vi "Current Channels Array.vi"(0 "Channel 1":string, 5 "Relays Array In":bool[](array[boolean])=[FALSE, FALSE, FALSE, FALSE, FALSE, FALSE, FALSE, FALSE, FALSE, FALSE, FALSE, FALSE, FALSE, FALSE, FALSE, FALSE, FALSE, FALSE, FALSE, FALSE, FALSE, FALSE, FALSE, FALSE, FALSE, FALSE, FALSE, FALSE, FALSE, FALSE, FALSE, FALSE, FALSE, FALSE, FALSE, FALSE, FALSE, FALSE, FALSE, FALSE, FALSE, FALSE, FALSE, FALSE, FALSE, FALSE, FALSE, FALSE, FALSE, FALSE, FALSE, FALSE, FALSE, FALSE, FALSE, FALSE, FALSE, FALSE, FALSE, FALSE, FALSE, FALSE, FALSE, FALSE, FALSE, FALSE, FALSE, FALSE, FALSE, FALSE, FALSE, FALSE, FALSE, FALSE, FALSE, FALSE, FALSE, FALSE, FALSE, FALSE, FALSE, FALSE, FALSE, FALSE, FALSE, FALSE, FALSE, FALSE, FALSE, FALSE, FALSE, FALSE, FALSE, FALSE, FALSE, FALSE], 7 "N shift to Min Channel Current":u32, 9 "Range and Function":T1(ring), 11 "error in":errorcluster, 13 "State":bool) -> (4 "Current Channel?":bool, 6 "Relay Array out":bool[](array[boolean]), 15 "error out":errorcluster)   [LabVIEW 2021, in "DMM_Scan DAQ Ext RLY.lvlib"]
doc: "Checks if Channel 1 from the Scan List is a current channel and will Open/Close the corresponding Shunt Relay in the Relay Array."
uses:
  DMM_Scan DAQ Ext RLY.lvlib
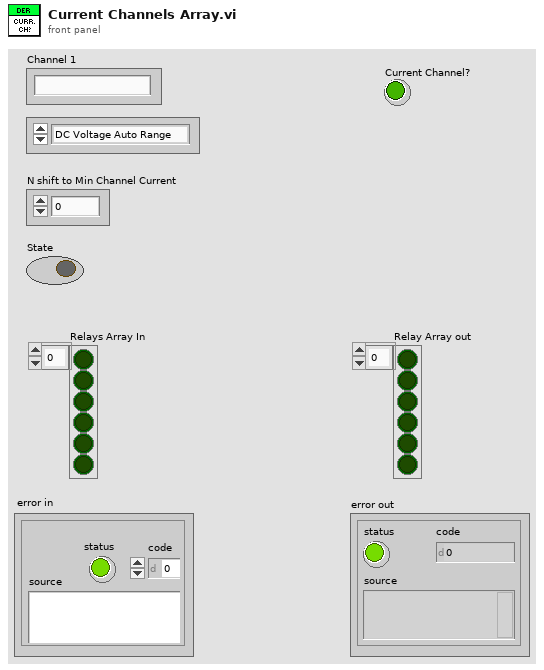
[diagram p1: front panel]
types:
  T1 = enum16{"DC Voltage Auto Range", "DC 100 mV", "DC 1 V ", "DC 10 V", "DC 100 V", "DC 300 V", " ", "AC Voltage Auto Range", "AC 50 mV", "AC 200 mV", "AC 500 mV", "AC 2 V", "AC 5 V", "AC 20 V", "AC 50 V", "AC 300 V", "  ", "DC Current Auto Range", "DC 1 uA", "DC 10 uA", "DC 100 uA", "DC 1 mA", "DC 10 mA", "DC 20 mA", "DC 100 mA", "DC 200 mA", "DC 1 A", "DC 3 A", "   ", "AC Current Auto Range", "AC 100 uA", "AC 1 mA", "AC 10 mA", "AC 100 mA", "AC 500 mA", "AC 1 A", "AC 3 A", "    ", "Resistance Auto Range", "Res 100 Ohm", "Res 1 kOhm", "Res 10 kOhm", "Res 100 kOhm", "Res 1 MOhm", "Res 10 MOhm", "Res 100 MOhm", "Res 5 GOhm", "     ", "Frequency AC Auto Range", "Freq AC 50 mV", "Freq AC 500 mV", "Freq AC 5 V", "Freq AC 50 V", "Freq AC 300 V", "      ", "Period AC Auto Range", "Period AC 50 mV", "Period AC 500 mV", "Period AC 5 V", "Period AC 50 V", "Period AC 300 V"}
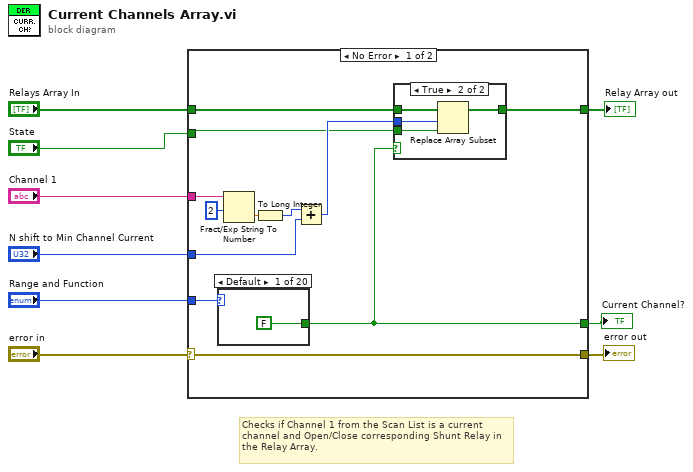
[diagram p0: block diagram]
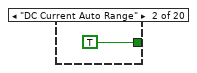
[diagram p3: hidden frame]
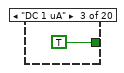
[diagram p4: hidden frame]
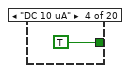
[diagram p5: hidden frame]
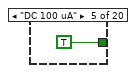
[diagram p6: hidden frame]
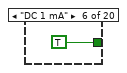
[diagram p7: hidden frame]
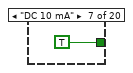
[diagram p8: hidden frame]
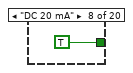
[diagram p9: hidden frame]
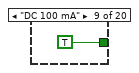
[diagram p10: hidden frame]
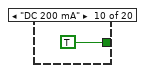
[diagram p11: hidden frame]
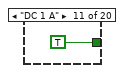
[diagram p12: hidden frame]
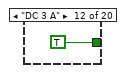
[diagram p13: hidden frame]
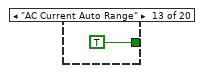
[diagram p14: hidden frame]
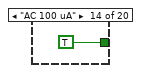
[diagram p15: hidden frame]
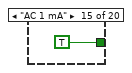
[diagram p16: hidden frame]
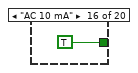
[diagram p17: hidden frame]
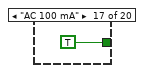
[diagram p18: hidden frame]
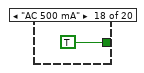
[diagram p19: hidden frame]
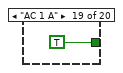
[diagram p20: hidden frame]
diagram:
  # "Checks if Channel 1 from the Scan List is a current channel and Open/Close corresponding Shunt Relay in the Relay Array."
  n1 = case shown="No Error" "error in" {
    selector: "error in" -> [w19 w49]
    tunnel: "Channel 1" -> [w17 _]
    tunnel: [w19 w49] -> w7
    tunnel: [w10 FALSE] -> w6
    tunnel: "N shift to Min Channel Current" -> [w16 _]
    tunnel: "Relays Array In" -> [w13 w47]
    tunnel: [w15 w47] -> w3
    tunnel: "State" -> [w12 _]
    tunnel: "Range and Function" -> [w11 _]
    frame No Error {
      n2 = case shown="Default" w11 {
        tunnel: [FALSE TRUE TRUE TRUE TRUE TRUE TRUE TRUE TRUE TRUE TRUE TRUE TRUE TRUE TRUE TRUE TRUE TRUE TRUE TRUE] -> w10
        frame Default {
        }
        frame "DC Current Auto Range" {
        }
        frame "DC 1 uA" {
        }
        frame "DC 10 uA" {
        }
        frame "DC 100 uA" {
        }
        frame "DC 1 mA" {
        }
        frame "DC 10 mA" {
        }
        frame "DC 20 mA" {
        }
        frame "DC 100 mA" {
        }
        frame "DC 200 mA" {
        }
        frame "DC 1 A" {
        }
        frame "DC 3 A" {
        }
        frame "AC Current Auto Range" {
        }
        frame "AC 100 uA" {
        }
        frame "AC 1 mA" {
        }
        frame "AC 10 mA" {
        }
        frame "AC 100 mA" {
        }
        frame "AC 500 mA" {
        }
        frame "AC 1 A" {
        }
        frame "AC 3 A" {
        }
      }
      n3 = Fract/Exp String To Number(string=w17, offset=2 ("offset (0)")) -> (number=w20:dbl)  [unwired: 2 in, 1 out]
      n4 = To Long Integer(number=w20) -> (32bit integer=w18:i32)
      n5 = Add(x=w18, y=w16) -> (x+y=w14:u32)
      n6 = case shown="True" w10 {
        tunnel: [w22 w26] -> w15
        tunnel: w14 -> [_ w25]
        tunnel: w13 -> [w22 w24]
        tunnel: w12 -> [_ w23]
        frame False {
        }
        frame True {
          n7 = Replace Array Subset(array=w24, new element=w23, index=w25) -> (w26:bool[])
        }
      }
    }
    frame Error {
    }
  }
  "error out" <- w7
  "Current Channel?" <- w6
  "Relay Array out" <- w3
